vi "Save2ColorPNG.vi"(6 "Time Stamp?":bool=TRUE, 7 "File Name Prefix":string="ns_FLIM", 8 "error in":errorcluster, 9 "Identify Name":string="Mix_Phase0", 10 "Data Picture":picture, 11 "Parent Directory":path) -> (0 "error out":errorcluster, 3 "cancelled":bool)   [LabVIEW 2015]
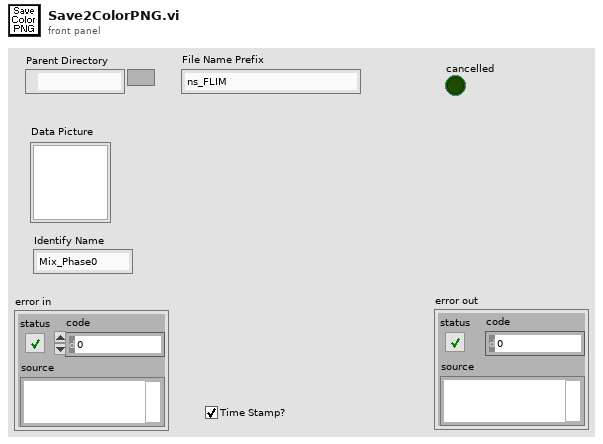
[diagram p1: front panel]
types:
  T1 = enum16{"open", "replace", "create", "open or create", "replace or create", "replace or create with confirmation"}
  T2 = typedef "imagedata.ctl" = cluster{"image type":i32, "image depth":i32, "image":u8[], "mask":u8[], "colors":u32[], "Rectangle":cluster{"left":i16, "top":i16, "right":i16, "bottom":i16}}
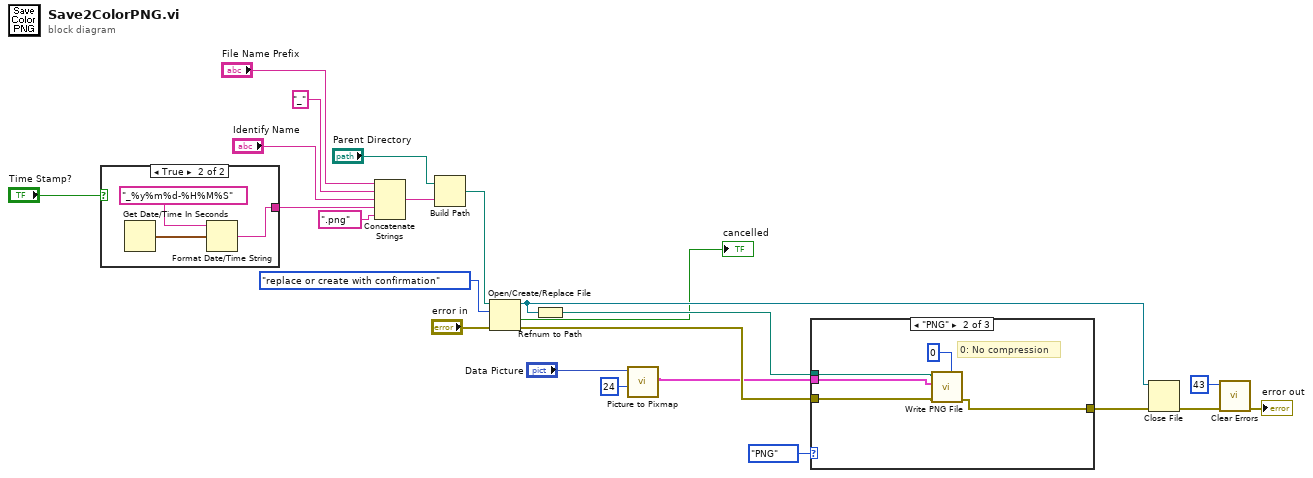
[diagram p0: block diagram]
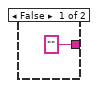
[diagram p2: hidden frame]
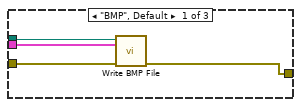
[diagram p3: hidden frame]
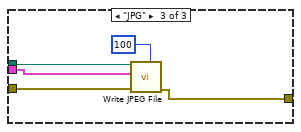
[diagram p4: hidden frame]
diagram:
  n1 = case shown="True" "Time Stamp?" {
    tunnel: ["" w25] -> w2
    frame False {
    }
    frame True {
      n2 = Get Date/Time In Seconds() -> (seconds since 1Jan1904=w26:timestamp)
      n3 = Format Date/Time String(time format string (%c)="_%y%m%d-%H%M%S", seconds (now)=w26) -> (date/time string=w25:string)  [unwired: 1 in]
    }
  }
  n4 = Concatenate Strings("File Name Prefix", "_" ("string"), "Identify Name", w2, ".png" ("string")) -> (w23:string)
  n5 = Build Path(base path="Parent Directory", name or relative path=w23) -> (appended path=w16:path)
  n6 = Open/Create/Replace File(file path (use dialog)=w16, error in="error in", operation (0:open)=T1."replace or create with confirmation") -> (refnum out=w11:refnum<file>, cancelled=→"cancelled":bool, error out=w9:errorcluster)  [unwired: 3 in]
  n7 = Refnum to Path(1:w11) -> (0:w10:path)
  n8 = call <vilib>:"Picture to Pixmap.vi"("depth"=24, "picture"="Data Picture") -> ("image data"=w4:T2)  [unwired: 8 in, 1 out]
  n9 = case shown="\"PNG\"" enum16{"BMP", "PNG", "JPG"}."PNG" {
    tunnel: w10 -> [w28 w33 w37]
    tunnel: w4 -> [w29 w34 w38]
    tunnel: w9 -> [w31 w36 w40]
    tunnel: [w30 w35 w39] -> w8
    frame "BMP", Default {
      n10 = call <vilib>:"Write BMP File.vi"("error in (no error)"=w31, "image data"=w29, "path to BMP file"=w28) -> ("error out"=w30:errorcluster)  [unwired: 7 in, 1 out]
    }
    frame "PNG" {
      # "0: No compression"
      n11 = call <vilib>:"Write PNG File.vi"("compression (default)"=0, "error in (no error)"=w36, "image data"=w34, "path to PNG file"=w33) -> ("error out"=w35:errorcluster)  [unwired: 6 in, 1 out]
    }
    frame "JPG" {
      n12 = call <vilib>:"Write JPEG File.vi"("quality (80)"=100, "error in (no error)"=w40, "image data"=w38, "path to JPEG file"=w37) -> ("error out"=w39:errorcluster)  [unwired: 6 in, 1 out]
    }
  }
  n13 = Close File(refnum=w11, error in=w8) -> (error out=w12:errorcluster)  [unwired: 1 out]
  n14 = call <vilib>:"Clear Errors.vi"("error in (no error)"=w12, "specific error code to clear (0: all)"=43) -> ("error out"=→"error out":errorcluster)  [unwired: 4 in, 1 out]
